vi "RequestControl.vi"(8 "error in (no error)":errorcluster, 9 "level in":T1, 10 "who wants?":string, 11 "BME_DG_System in":refnum<class "BME_DG_System.lvclass">) -> (0 "error out":errorcluster, 1 "level out":T1, 2 "locked by out":string, 3 "BME_DG_System out":refnum<class "BME_DG_System.lvclass">, 5 "Success?":bool)   [LabVIEW 2009, in "POLARIS BME DG.lvlib" / "BME_DG_System.lvclass"]
doc: "This VI is usefull for systems with slow repeteation rate like POLARIS laser system.\n\nIn sync mode the channel delay values will be set also syncronuosly, it is not practical for round trip alagnment times of regenative amplifiers, because we have to wait till slowest channel fires until parameter change. In reason to avoid this problem two control mode have been defined:\n\n- simple: for channel delay changes\n- expert: for output modulo changes\n\nin simple mode the sync bit of master channels is deaktivated and asynchron parameter updates occures. In expert mode, the bit is true, so sync mode is activate."
uses:
  BME_DG_System.lvclass
  ControlLevel.ctl
  BME_DG_System.lvclass/BME_DG_System.ctl
  POLARIS BME DG.lvlib
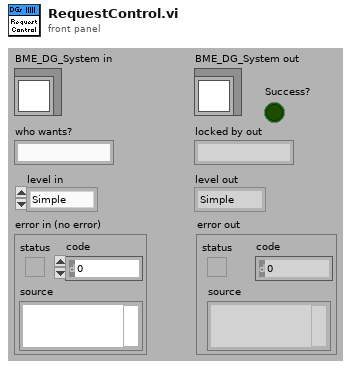
[diagram p1: front panel]
types:
  T1 = typedef "POLARIS BME DG.lvlib/BME_DG_System.lvclass/ControlLevel.ctl" = enum16{"Simple", "Expert", "Unknown"}
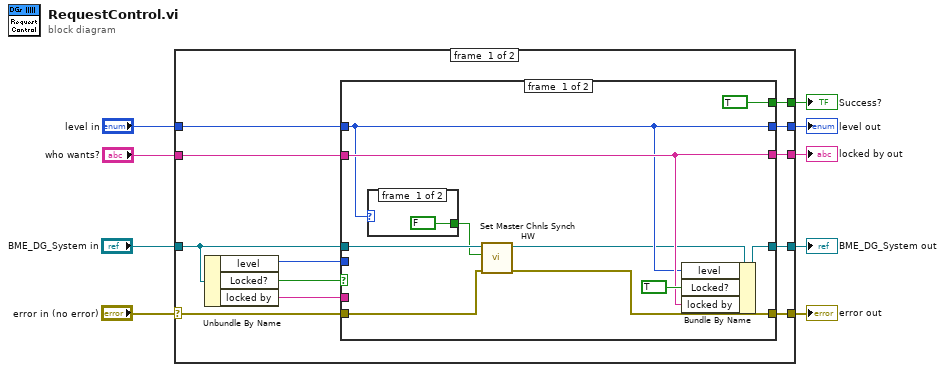
[diagram p0: block diagram]
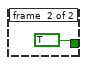
[diagram p2: hidden frame]
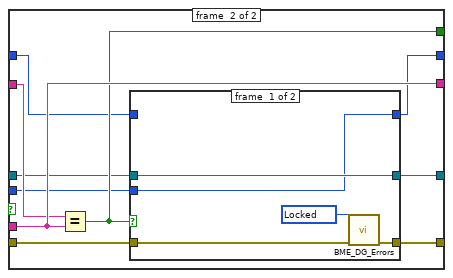
[diagram p3: hidden frame]
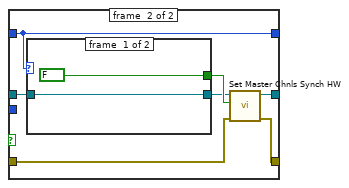
[diagram p4: hidden frame]
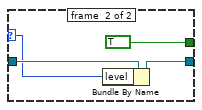
[diagram p5: hidden frame]
diagram:
  n1 = case shown="No Error" "error in (no error)" {
    selector: "error in (no error)" -> [w19 w63]
    tunnel: [w18 w63] -> w8
    tunnel: [w17 w62] -> w6
    tunnel: "BME_DG_System in" -> [w16 w62]
    tunnel: [w15 _] -> w5
    tunnel: [w14 _] -> w4
    tunnel: [w13 _] -> w3
    tunnel: "level in" -> [w12 _]
    tunnel: "who wants?" -> [w10 _]
    frame #0 {
      n2 = Unbundle By Name(w16) -> ("level"=w11:T1, "Locked?"=w21:bool, "locked by"=w20:string)
      n3 = case shown="True" w21 {
        tunnel: w20 -> [_ w41]
        tunnel: w19 -> [w24 w43]
        tunnel: [w23 w42] -> w18
        tunnel: [w31 w37] -> w17
        tunnel: w16 -> [w26 w38]
        tunnel: [w28 w41] -> w15
        tunnel: [TRUE w39] -> w14
        tunnel: [w27 w35] -> w13
        tunnel: w12 -> [w27 w36]
        tunnel: w11 -> [_ w34]
        tunnel: w10 -> [w28 w40]
        frame #0 {
          n4 = case shown="\"Expert\", Default" w27 {
            tunnel: [FALSE ("Locked?") TRUE ("Locked?")] -> w22
            frame #0 {
            }
            frame #1 {
            }
          }
          n5 = call-dynamic "Set Master Chnls Synch HW.vi"("error in (no error)"=w24, "Synch?"=w22, "BME_DG_System in"=w26) -> ("error out"=w23:errorcluster, "BME_DG_System out"=w25:refnum<class "BME_DG_System.lvclass">)  [unwired: 7 in]
          n6 = Bundle By Name(cluster=w25, "level"=w27, "Locked?"=TRUE, "locked by"=w28) -> (w31:refnum<class "BME_DG_System.lvclass">)
        }
        frame #1 {
          n7 = Equal?(x=w40, y=w41) -> (x = y?=w39:bool)
          n8 = case shown="False" w39 {
            tunnel: w43 -> [w48 w54]
            tunnel: [w47 w53] -> w42
            tunnel: w38 -> [w45 w50]
            tunnel: [w45 w55] -> w37
            tunnel: w36 -> [_ w51]
            tunnel: [w44 w51] -> w35
            tunnel: w34 -> [w44 _]
            frame #0 {
              w46 = 503013 items=["Channel refers itself"=503001, "Deadloop"=503002, "Negative Delay"=503003, "Delay Card not found"=503004, "Channel not found"=503005, "Parse Error"=503006, "Not Supported"=503007, "Systen not found"=503008, "To much masters"=503009, "None master in Syterm"=503010, "InterruptError"=503011, "ChnlPeriodeWarning"=503012, "Locked"=503013] ("error")
              n9 = call "BME_DG_Errors.vi"("error in (no error)"=w48, "error"=w46) -> ("error out"=w47:errorcluster)  [unwired: 9 in]
            }
            frame #1 {
              n10 = case shown="\"Expert\", Default" w51 {
                selector: w51 -> [_ w58]
                tunnel: [FALSE ("Locked?") TRUE ("Locked?")] -> w52
                tunnel: w50 -> [w56 w60]
                tunnel: [w56 w59] -> w49
                frame #0 {
                }
                frame #1 {
                  n11 = Bundle By Name(cluster=w60, "level"=w58) -> (w59:refnum<class "BME_DG_System.lvclass">)
                }
              }
              n12 = call-dynamic "Set Master Chnls Synch HW.vi"("error in (no error)"=w54, "Synch?"=w52, "BME_DG_System in"=w49) -> ("error out"=w53:errorcluster, "BME_DG_System out"=w55:refnum<class "BME_DG_System.lvclass">)  [unwired: 7 in]
            }
          }
        }
      }
    }
    frame #1 {
    }
  }
  "error out" <- w8
  "BME_DG_System out" <- w6
  "locked by out" <- w5
  "Success?" <- w4
  "level out" <- w3
